vi "Initial Setting Zero Point.vi"(11 "output cluster":T1) -> ()   [LabVIEW 2016]
uses:
  Controls/Cal Refs.ctl
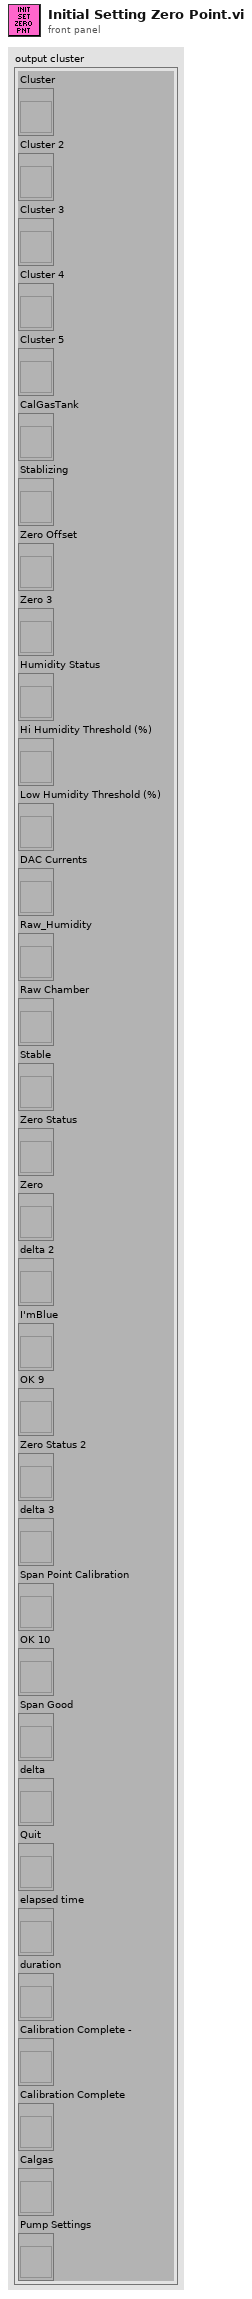
[diagram p1: front panel]
types:
  T1 = typedef "Cal Refs.ctl" = cluster{"Cluster":refnum<vi>, "Cluster 2":refnum<vi>, "Cluster 3":refnum<vi>, "Cluster 4":refnum<vi>, "Cluster 5":refnum<vi>, "CalGasTank":refnum<vi>, "Stablizing":refnum<vi>, "Zero Offset":refnum<vi>, "Zero 3":refnum<vi>, "Humidity Status":refnum<vi>, "Hi Humidity Threshold (%)":refnum<vi>, "Low Humidity Threshold (%)":refnum<vi>, "DAC Currents":refnum<vi>, "Raw_Humidity":refnum<vi>, "Raw Chamber":refnum<vi>, "Stable":refnum<vi>, "Zero Status":refnum<vi>, "Zero":refnum<vi>, "delta 2":refnum<vi>, "I'mBlue":refnum<vi>, "OK 9":refnum<vi>, "Zero Status 2":refnum<vi>, "delta 3":refnum<vi>, "Span Point Calibration":refnum<vi>, "OK 10":refnum<vi>, "Span Good":refnum<vi>, "delta":refnum<vi>, "Quit":refnum<vi>, "elapsed time":refnum<vi>, "duration":refnum<vi>, "Calibration Complete -":refnum<vi>, "Calibration Complete":refnum<vi>, "Calgas":refnum<vi>, "Pump Settings":refnum<vi>}
  T2 = enum16{"Setting Zero at 5 mA", "Setting Zero at 15 mA", "Calculating slopes"}
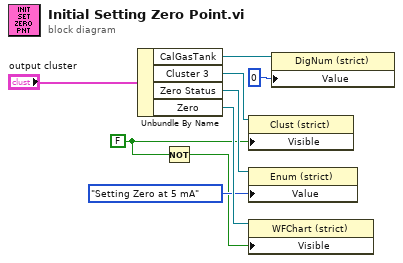
[diagram p0: block diagram]
diagram:
  w2 = FALSE ("Visible")
  n1 = Unbundle By Name("output cluster") -> ("CalGasTank"=w4:refnum<vi>, "Cluster 3"=w6:refnum<vi>, "Zero Status"=w7:refnum<vi>, "Zero"=w8:refnum<vi>)
  n2 = Not(x=w2) -> (.not. x?=w1:bool)
  n3 = property on="Property Node" class="Clust (strict)"(reference=w6, "Visible"=w2) -> ()  [unwired: 1 in, 2 out]
  n4 = property class="Enum (strict)"(reference=w7, "Value"=T2."Setting Zero at 5 mA" ("Zero Status")) -> ()  [unwired: 1 in, 2 out]
  n5 = property on="Property Node" class="WFChart (strict)"(reference=w8, "Visible"=w1) -> ()  [unwired: 1 in, 2 out]
  n6 = property class="DigNum (strict)"(reference=w4, "Value"=u8 0 ("CalGasTank")) -> ()  [unwired: 1 in, 2 out]
